vi "Untitled 1 (SubVI).vi"(10 "Numeric 3":dbl, 11 "Numeric 4":dbl) -> (3 "Numeric":dbl)   [LabVIEW 2018]
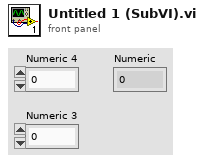
[diagram p1: front panel]
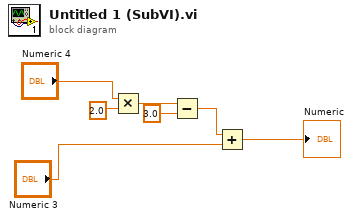
[diagram p0: block diagram]
diagram:
  n1 = Multiply(x="Numeric 4", y=2.0) -> (x*y=w1:dbl)
  n2 = Subtract(x=w1, y=3.0) -> (x-y=w3:dbl)
  n3 = Add(x=w3, y="Numeric 3") -> (x+y=→"Numeric":dbl)
